vi "Get_message_from_UI.vi"(11 "error in (no error)":errorcluster, 12 "timeout in ms (1000)":i32=1000) -> (4 "data DVR out":refnum<data-value>, 10 "output valid?":bool, 15 "error out":errorcluster)   [LabVIEW 2019, in "Service.lvlib"]
uses:
  Service.lvlib
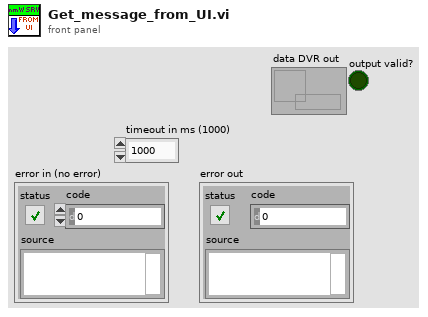
[diagram p1: front panel]
types:
  T1 = typedef "Service.lvlib/AppData.ctl" = cluster{"MsgQ":refnum<queue>, "Stop?":bool, "zmq sessions":cluster{"Control_endpoint":string, "Instr_endpoint":string}, "control-loop":cluster{"fromUI-Q":refnum<queue>, "toUI":refnum<user-event>, "Control_endpoint":string}, "UI-loop":cluster{"evnt_ref":refnum<event-registration>}, "logging":cluster{"level":dbl, "verbosity":dbl, "path":string, "Listener_ID":string}, "general_settings":cluster{"mmW_instr_ini_path":string, "mmW_instr_pid_path":string}}
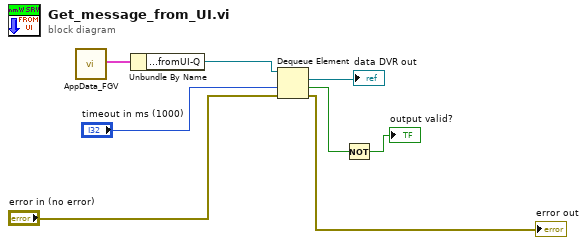
[diagram p0: block diagram]
diagram:
  n1 = call "AppData_FGV.vi"() -> ("AppData out"=w8:T1)  [unwired: 18 in, 1 out]
  n2 = Unbundle By Name(w8) -> ("control-loop.fromUI-Q"=w7:refnum<queue>)
  n3 = Dequeue Element(queue=w7, timeout in ms (-1)="timeout in ms (1000)", error in (no error)="error in (no error)") -> (element=→"data DVR out":refnum<data-value>, timed out?=w2:bool, error out=→"error out":errorcluster)  [unwired: 1 out]
  n4 = Not(x=w2) -> (.not. x?=→"output valid?":bool)
